vi "GetSetBlackLevelAuto.vi"(7 "Set?":bool, 8 "error in (no error)":errorcluster, 10 "Value in":T1, 11 "Camera in":refnum<class "Camera.lvclass">) -> (0 "error out":errorcluster, 2 "Value out":T1)   [LabVIEW 2020, in "Camera.lvclass"]
uses:
  Camera.lvclass
  Camera.lvclass/Camera.ctl
  bin/gindustrialcam_32-1.dll
  Auto Mode.ctl
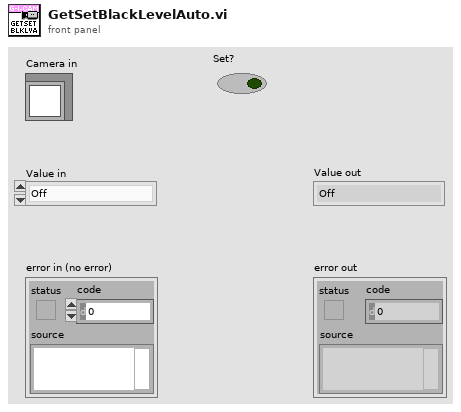
[diagram p1: front panel]
types:
  T1 = typedef "Camera.lvclass/Auto Mode.ctl" = enum8{"Off", "Once", "Continuous"}
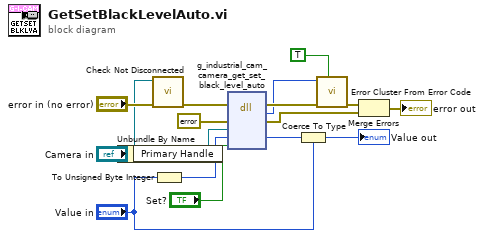
[diagram p0: block diagram]
diagram:
  n1 = Unbundle By Name("Camera in") -> ("Primary Handle"=w7:refnum<data-value>)
  n2 = call "Check Not Disconnected.vi"("error in (no error)"="error in (no error)", "Camera in"="Camera in") -> ("error out"=w2:errorcluster)  [unwired: 9 in]
  n3 = To Unsigned Byte Integer(number="Value in") -> (unsigned 8bit integer=w6:u8)
  n4 = dll-call lib="C:/serenial/lib/g-industrial-camera/LabVIEW/g_industrial_cam/bin/gindustrialcam_*-1.*" fn="g_industrial_cam_camera_get_set_black_level_auto"(error in=w2, "err"=errorcluster {"status"=FALSE, "code"=0, "source"=""} ("error constant"), "edvr"=w7, "value"=w6, "set"="Set?") -> (error out=w16:errorcluster, "Mg_Error"=w15:i32, "err"=w13:errorcluster, "value"=w5:u8)  [unwired: 4 in, 1 out]
  n5 = Coerce To Type(0:w5, 1:"Value in") -> (2:→"Value out":T1)
  n6 = call <vilib>:"Error Cluster From Error Code.vi"("show call chain? (False)"=TRUE, "error in (no error)"=w16, "error code (0)"=w15) -> ("error out"=w14:errorcluster)  [unwired: 6 in]
  n7 = Merge Errors(w14, w13) -> (→"error out":errorcluster)
